vi "Get Libraries Names and Paths.vi"(8 "error in":errorcluster, 11 "Project in":refnum<class "Project.lvclass">) -> (0 "error out":errorcluster, 3 "Project out":refnum<class "Project.lvclass">)   [LabVIEW 2020, in "Panther Dashboard.lvlib" / "Project.lvclass"]
uses:
  Project.lvclass
  Project.lvclass/Project.ctl
  LabVIEWItem/LabVIEWItem.lvclass/LabVIEWItem.ctl
  LabVIEWItem/Read Item Name.vi
  LabVIEWItem/Read Item Path.vi
  Read Libraries.vi
  Library/Library.lvclass
  C:/GitClones/PantherDashboard/src/LabVIEW/Panther Dashboard/Class/LabVIEWItem/LabVIEWItem.lvclass
panel:
  out "Libraries Paths":path[](array[path])
  out "Libraries Names":string[](array[string])
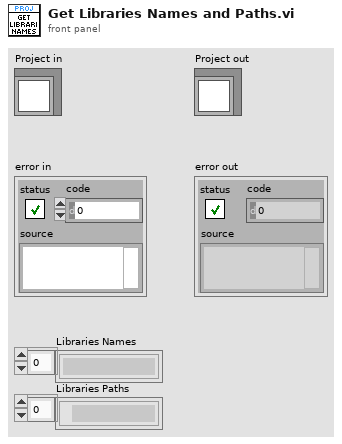
[diagram p1: front panel]
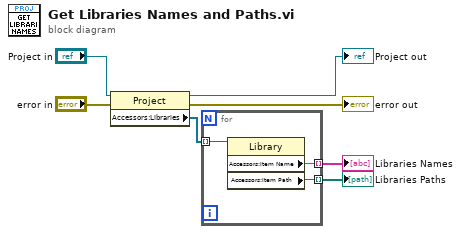
[diagram p0: block diagram]
diagram:
  n1 = property class="Project"(reference="Project in", error in="error in") -> (reference out=→"Project out":refnum<class "Project.lvclass">, error out=→"error out":errorcluster, "Accessors:Libraries"=w3:refnum<class "Library.lvclass">[])
  n2 = for {
    tunnel: w3 -> [w10] mode=indexing
    tunnel: [w9] -> w2 mode=indexing
    tunnel: [w8] -> w1 mode=indexing
    n3 = property class="Library"(reference=w10) -> ("Accessors:Item Name"=w9:string, "Accessors:Item Path"=w8:path)  [unwired: 1 in, 2 out]
  }
  "Libraries Names" <- w2
  "Libraries Paths" <- w1
